vi "Initialize.vi"(8 "error in (no error)":errorcluster, 11 "NXP LPCXpresso54608 in":refnum<class "NXP LPCXpresso54608.lvclass">) -> (0 "error out":errorcluster, 2 "Connected?":bool, 3 "NXP LPCXpresso54608 out":refnum<class "NXP LPCXpresso54608.lvclass">)   [LabVIEW 2020, in "NXP LPCXpresso54608.lvclass"]
doc: "Initialize a device."
uses:
  NXP LPCXpresso54608.lvclass
  MCU/MCU.lvclass
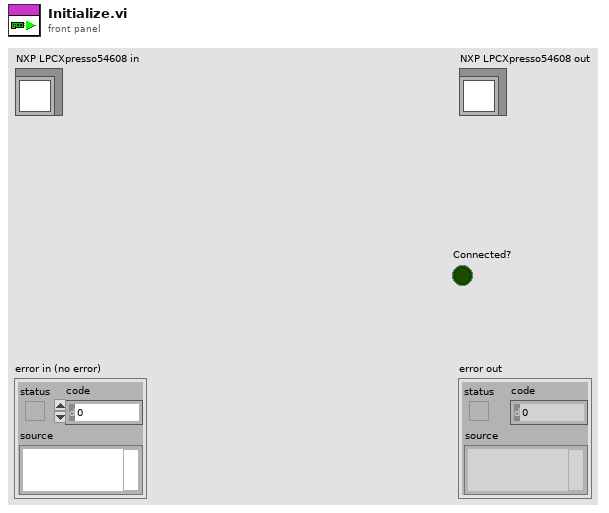
[diagram p1: front panel]
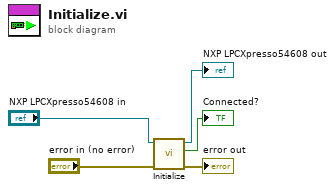
[diagram p0: block diagram]
diagram:
  n1 = call-parent "Initialize.vi"("error in (no error)"="error in (no error)", "MCU in"="NXP LPCXpresso54608 in") -> ("error out"=→"error out":errorcluster, "Connected?"=→"Connected?":bool, "MCU out"=→"NXP LPCXpresso54608 out":refnum<class "NXP LPCXpresso54608.lvclass">)  [unwired: 7 in]
